vi "Close.vi"(8 "error in (no error)":errorcluster, 11 "Measurement2D in":refnum<class "Measurement2D.lvclass">) -> (0 "error out":errorcluster, 3 "Measurement2D out":refnum<class "Measurement2D.lvclass">)   [LabVIEW 2014, in "Measurement2D.lvclass"]
uses:
  Measurement2D.lvclass
  Instrument/Instrument/Instrument.lvclass
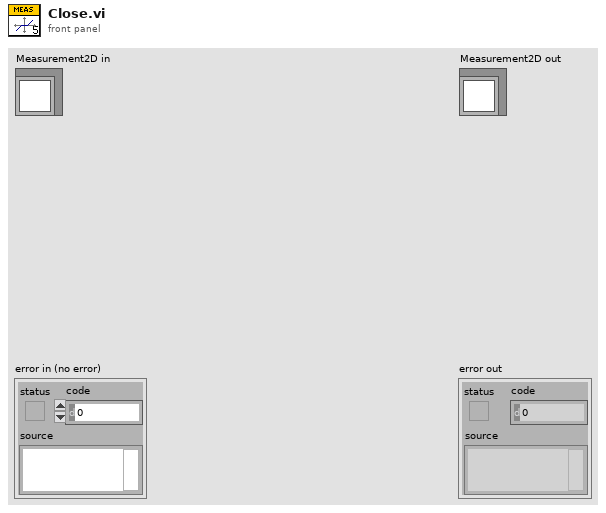
[diagram p1: front panel]
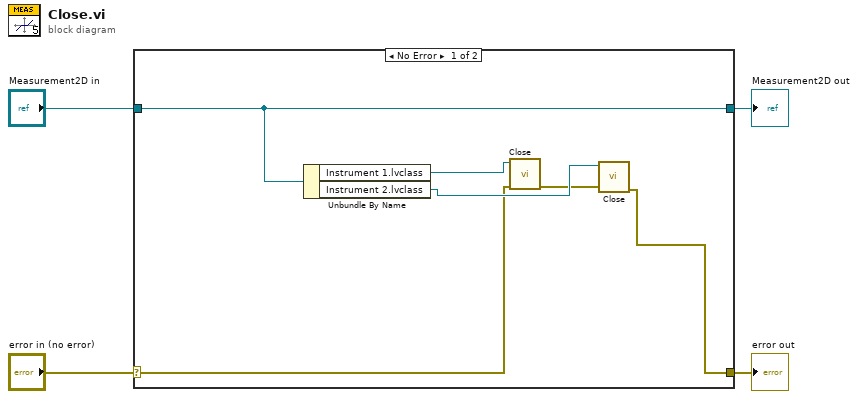
[diagram p0: block diagram]
diagram:
  n1 = case shown="No Error" "error in (no error)" {
    selector: "error in (no error)" -> [w6 w12]
    tunnel: [w5 w12] -> w3
    tunnel: [w10 w11] -> w1
    tunnel: "Measurement2D in" -> [w10 w11]
    frame No Error {
      n2 = Unbundle By Name(w10) -> ("Instrument 1.lvclass"=w9:refnum<class "Instrument.lvclass">, "Instrument 2.lvclass"=w8:refnum<class "Instrument.lvclass">)
      n3 = call-dynamic "Close.vi"("error in (no error)"=w6, "Instrument in"=w9) -> ("error out"=w7:errorcluster)  [unwired: 8 in, 1 out]
      n4 = call-dynamic "Close.vi"("error in (no error)"=w7, "Instrument in"=w8) -> ("error out"=w5:errorcluster)  [unwired: 8 in, 1 out]
    }
    frame Error {
    }
  }
  "error out" <- w3
  "Measurement2D out" <- w1
